vi "Logging_Using_MySQL.vi"() -> ()   [LabVIEW 2016]
uses:
  <vilib>/NI/Current Value Table/DataTypes/U16_Read.vi
  <vilib>/NI/Current Value Table/DataTypes/Boolean_Read.vi
  <vilib>/NI/Current Value Table/Type to Enum.vi
  <vilib>/NI/Current Value Table/DataTypes/U16_Type To Enum.vi
  <vilib>/NI/Current Value Table/DataTypes/Boolean_Type To Enum.vi
  <vilib>/Utility/file.llb/Read Delimited Spreadsheet (string).vi
  <vilib>/NI/Current Value Table/FGVs/CVT Globals.vi
  <vilib>/NI/Current Value Table/FGVs/Tag Memory.vi
  <vilib>/NI/Current Value Table/Memory Block.vi
  <vilib>/NI/Current Value Table/DataTypes/U16_Memory Block.vi
  <vilib>/NI/Current Value Table/DataTypes/Boolean_Memory Block.vi
  <vilib>/NI/Current Value Table/Current Value Table.lvlib
panel:
  out "Array":string[](array[string])
  out "error out 3":errorcluster
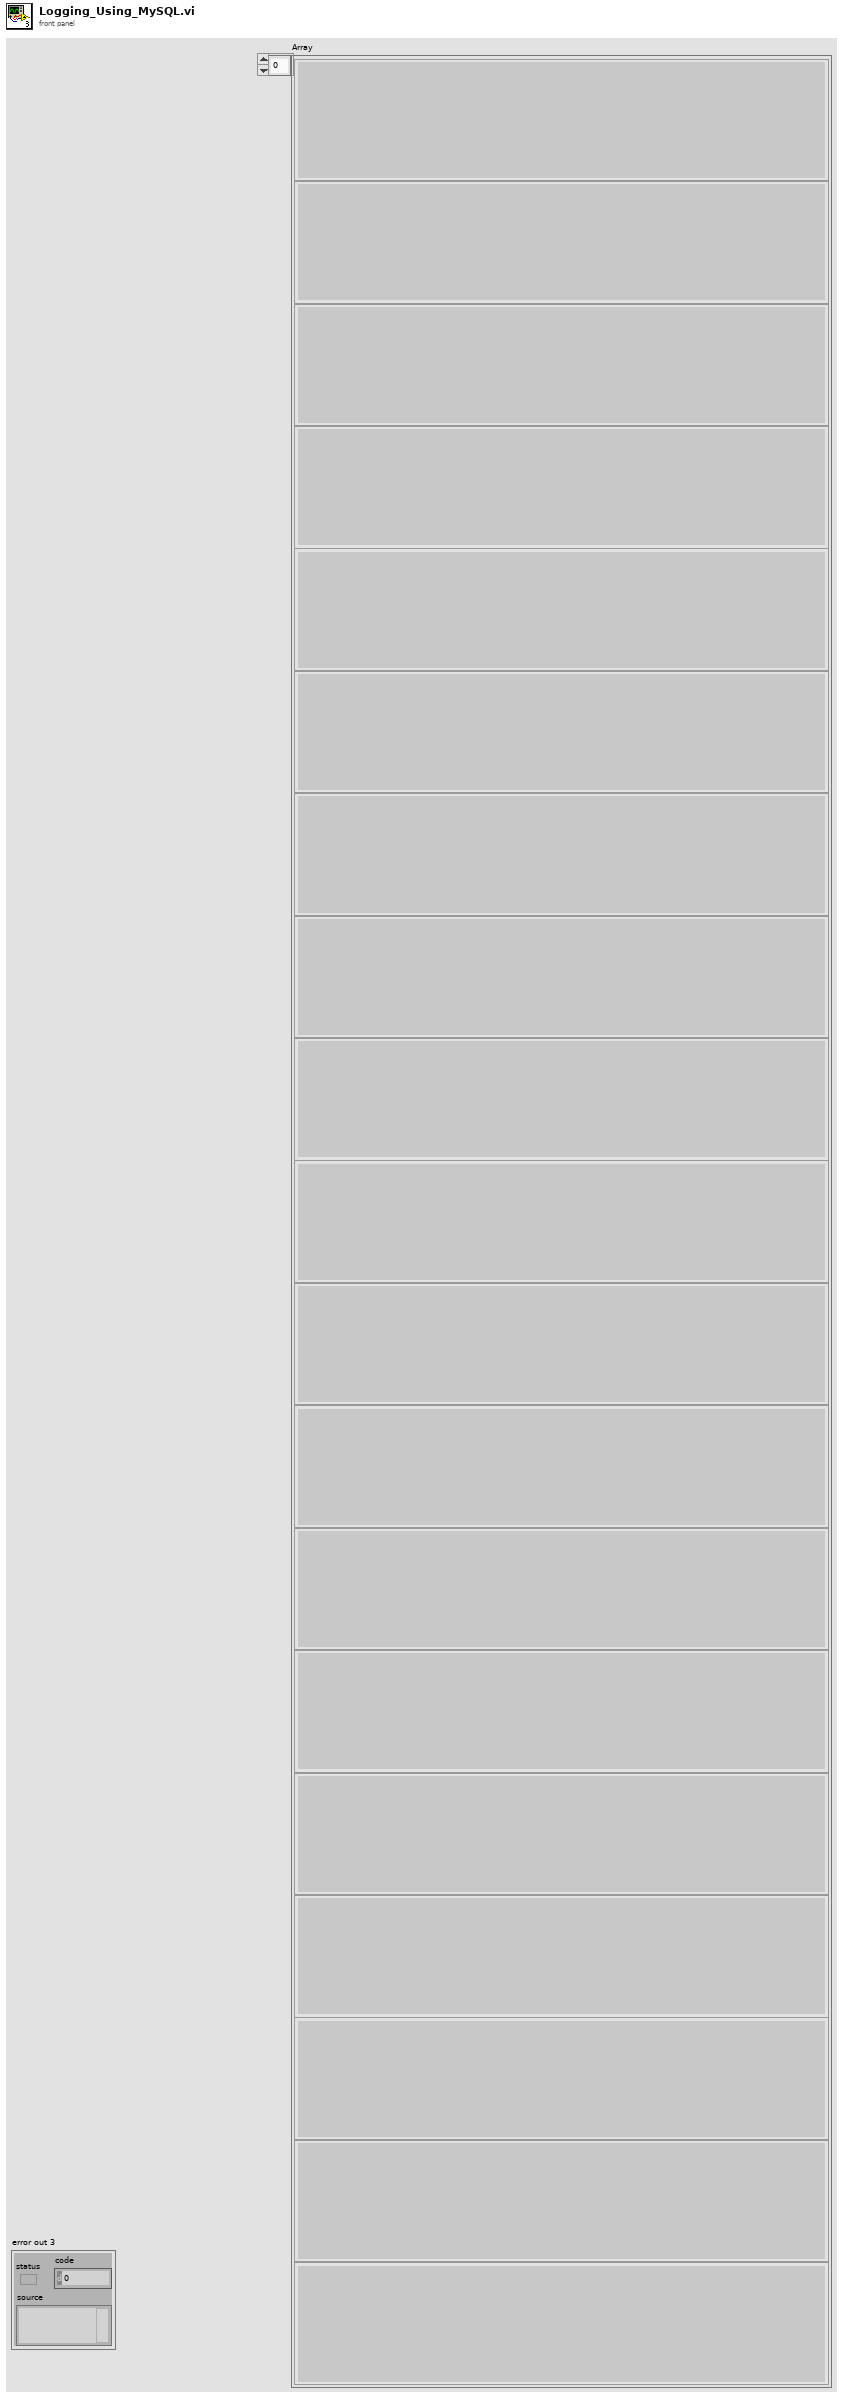
[diagram p1: front panel]
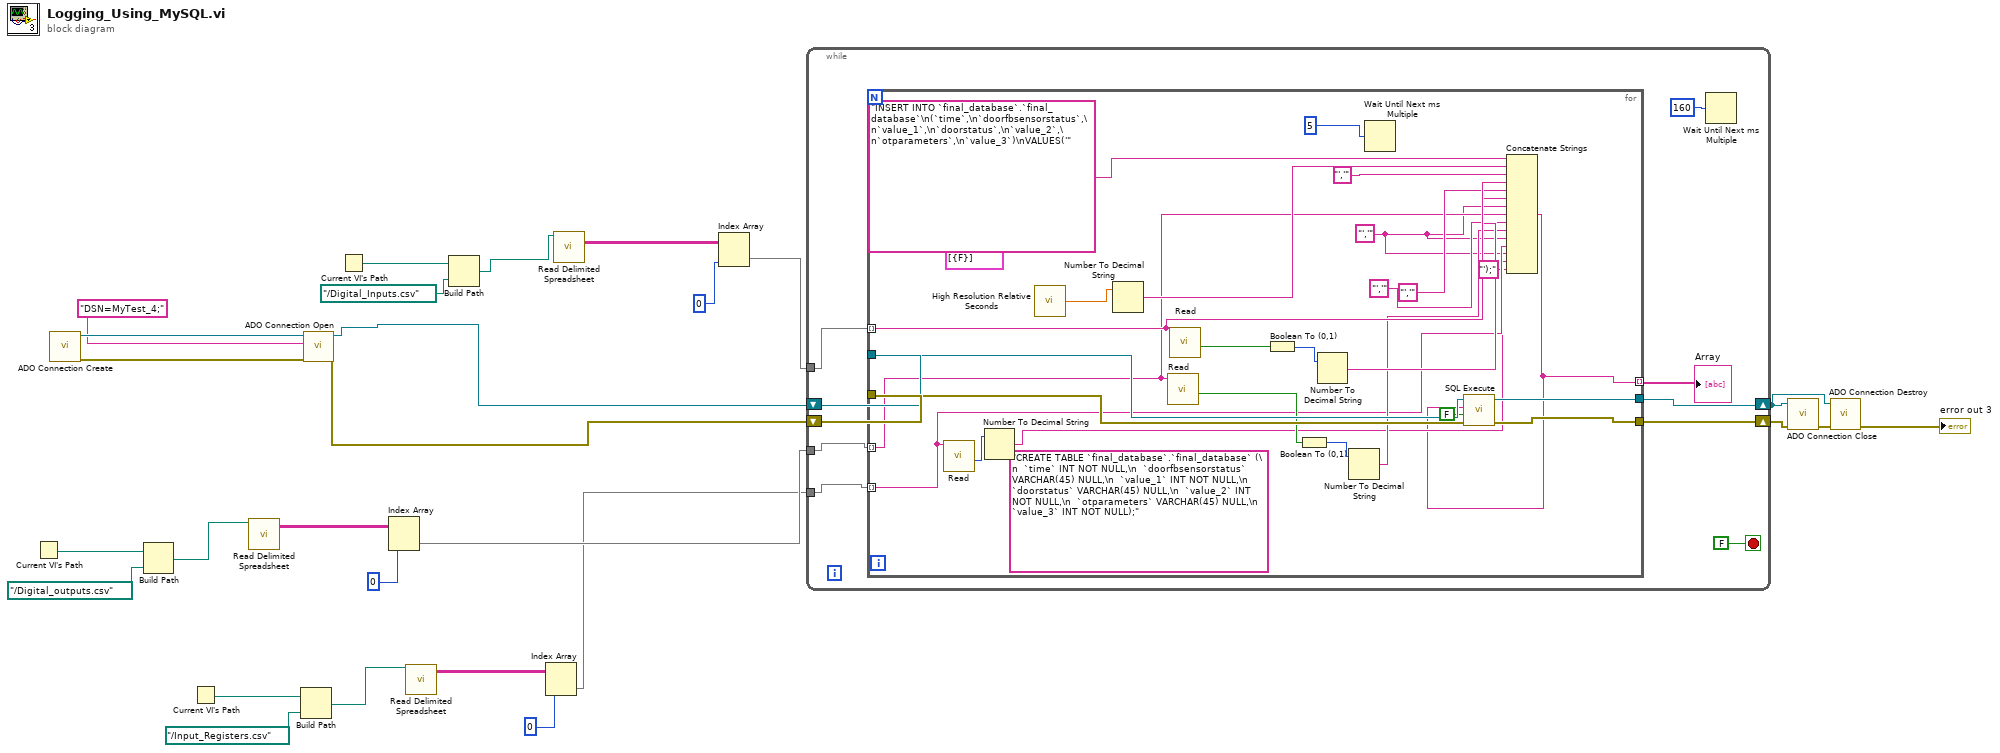
[diagram p0: block diagram]
diagram:
  n1 = Current VI's Path() -> (path=w12:path)
  n2 = call "ADO Connection Create.vi"() -> ("error out"=w20:errorcluster, "ADODB._Connection Out"=w21:refnum<k7>)  [unwired: 10 in]
  n3 = Build Path(base path=w12, name or relative path=path "../Digital_outputs.csv") -> (appended path=w11:path)
  n4 = Current VI's Path() -> (path=w6:path)
  n5 = call-poly <vilib>:"Read Delimited Spreadsheet.vi"("file path (dialog if empty)"=w11) -> ("all rows"=w10:string[][])  [unwired: 9 in, 5 out]
  n6 = Build Path(base path=w6, name or relative path=path "../Input_Registers.csv") -> (appended path=w5:path)
  n7 = call "ADO Connection Open.vi"("error in (no error)"=w20, "ConnectionString"="DSN=MyTest_4;" ("ConnectionString 2"), "ADODB._Connection In"=w21) -> ("error out"=w15:errorcluster, "ADODB._Connection Out"=w14:refnum<k7>)  [unwired: 7 in]
  n8 = Current VI's Path() -> (path=w24:path)
  n9 = Index Array(array=w10, index (col)=0 ("disabled index (col)")) -> (element=w8:string[])  [unwired: 1 in]
  n10 = call-poly <vilib>:"Read Delimited Spreadsheet.vi"("file path (dialog if empty)"=w5) -> ("all rows"=w4:string[][])  [unwired: 9 in, 5 out]
  n11 = Build Path(base path=w24, name or relative path=path "../Digital_Inputs.csv") -> (appended path=w22:path)
  n12 = Index Array(array=w4, index (col)=0 ("disabled index (col)")) -> (element=w1:string[])  [unwired: 1 in]
  n13 = call-poly <vilib>:"Read Delimited Spreadsheet.vi"("file path (dialog if empty)"=w22) -> ("all rows"=w26:string[][])  [unwired: 9 in, 5 out]
  n14 = Index Array "Index Array"(array=w26, index (col)=0 ("disabled index (col)")) -> (element=w25:string[])  [unwired: 1 in]
  n15 = while {
    tunnel: w25 -> [w37]
    shift-right: [w35] -> w16
    shift-left: w15 -> [w34]
    shift-right: [w32] -> w13
    shift-left: w14 -> [w33]
    tunnel: w8 -> [w29]
    tunnel: w1 -> [w28]
    stop <- FALSE stop-if-true
    (unwired) cluster{"Boolean":bool}[] [{"Boolean"=FALSE}] ("output array")
    n16 = for {
      tunnel: w37 -> [w55] mode=indexing
      tunnel: [w63] -> w32
      tunnel: [w62] -> w35
      tunnel: w34 -> [w61]
      tunnel: w33 -> [w60]
      tunnel: [w38] -> w30 mode=indexing
      tunnel: w29 -> [w49] mode=indexing
      tunnel: w28 -> [w43] mode=indexing
      w42 = "','" ("string")
      (unwired) "CREATE TABLE `final_database`.`final_database` (\n  `time` INT NOT NULL,\n  `doorfbsensorstatus` VARCHAR(45) NULL,\n  `value_1` INT NOT NULL,\n  `doorstatus` VARCHAR(45) NULL,\n  `value_2` INT NOT NULL,\n  `otparameters` VARCHAR(45) NULL,\n  `value_3` INT NOT NULL);"
      n17 = call-poly <vilib>:"Read.vi"("Tag Name"=w43) -> ("Value"=w41:u16)  [unwired: 9 in, 1 out]
      n18 = Number To Decimal String(number=w41) -> (decimal integer string=w40:string)  [unwired: 1 in]
      n19 = call <vilib>:"High Resolution Relative Seconds.vi"() -> ("relative seconds"=w53:dbl)
      n20 = Number To Decimal String(number=w53) -> (decimal integer string=w57:string)  [unwired: 1 in]
      n21 = call-poly <vilib>:"Read.vi"("Tag Name"=w49) -> ("Value"=w46:bool)  [unwired: 9 in, 1 out]
      n22 = call-poly <vilib>:"Read.vi"("Tag Name"=w55) -> ("Value"=w51:bool)  [unwired: 9 in, 1 out]
      n23 = Boolean To (0,1)(Boolean=w51) -> (0, 1=w52:i16)
      n24 = Boolean To (0,1)(Boolean=w46) -> (0, 1=w47:i16)
      n25 = Number To Decimal String(number=w52) -> (decimal integer string=w50:string)  [unwired: 1 in]
      n26 = Number To Decimal String(number=w47) -> (decimal integer string=w45:string)  [unwired: 1 in]
      n27 = Wait Until Next ms Multiple(millisecond multiple=u32 5 ("millisecond timer value")) -> ()  [unwired: 1 out]
      n28 = Concatenate Strings("INSERT INTO `final_database`.`final_database`\n(`time`,\n`doorfbsensorstatus`,\n`value_1`,\n`doorstatus`,\n`value_2`,\n`otparameters`,\n`value_3`)\nVALUES('", w57, "','" ("string"), w55, "','" ("string"), w50, w42, w49, "','" ("string"), w45, w42, w43, w42, w40, "');" ("string")) -> (w38:string)
      n29 = call "SQL Execute.vi"("error in (no error)"=w61, "Return Data (T)"=FALSE, "Command Text"=w38, "ADODB._Connection In"=w60) -> ("error out"=w62:errorcluster, "ADODB._Connection Out"=w63:refnum<k7>)  [unwired: 4 in, 2 out]
    }
    "Array" <- w30
    n30 = Wait Until Next ms Multiple(millisecond multiple=u32 160) -> ()  [unwired: 1 out]
  }
  n31 = call "ADO Connection Close.vi"("error in (no error)"=w16, "ADODB._Connection In"=w13) -> ("error out"=w17:errorcluster)  [unwired: 8 in, 1 out]
  n32 = call "ADO Connection Destroy.vi"("error in (no error)"=w17, "ADODB._Connection In"=w13) -> ("error out"=→"error out 3":errorcluster)  [unwired: 9 in]
